vi "Move to Named Position (Sub VI).vi"(10 "named_position":T1, 11 "_num_axes":i32) -> (0 "error out":errorcluster)   [LabVIEW 2020, in "Manipulator.lvlib"]
uses:
  Manipulator.lvlib
  Settings/Named Position.ctl
  Manipulator-CLIDriver/Manipulator CLI Driver.lvlib
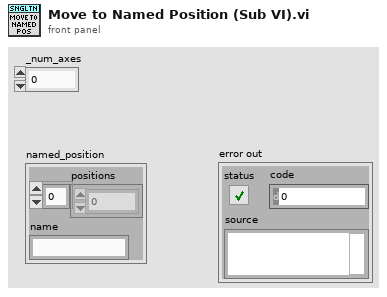
[diagram p1: front panel]
types:
  T1 = typedef "Manipulator.lvlib/Named Position.ctl" = cluster{"positions":dbl[], "name":string}
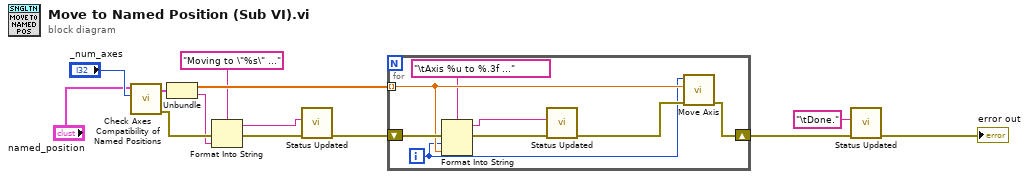
[diagram p0: block diagram]
diagram:
  n1 = call "Check Axes Compatibility of Named Positions.vi"("Num Axes"="_num_axes", "named_position"="named_position") -> ("error out"=w12:errorcluster, "named_position"=w11:T1)  [unwired: 8 in]
  n2 = Unbundle(w11) -> ("positions"=w8:dbl[], "name"=w4:string)
  n3 = Format Into String(format string="Moving to \"%s\" ...", error in=w12, w4) -> (resulting string=w5:string, error out=w7:errorcluster)  [unwired: 1 in]
  n4 = call "Status Updated.vi"("error in (no error)"=w7, "Status"=w5) -> ("error out"=w6:errorcluster)  [unwired: 9 in]
  n5 = for {
    tunnel: w8 -> [w16] mode=indexing
    shift-right: [w21] -> w9
    shift-left: w6 -> [w20]
    i -> [w15]
    n6 = Format Into String(format string="\tAxis %u to %.3f ...", error in=w20, w15, w16) -> (resulting string=w17:string, error out=w19:errorcluster)  [unwired: 1 in]
    n7 = call "Status Updated.vi"("error in (no error)"=w19, "Status"=w17) -> ("error out"=w18:errorcluster)  [unwired: 9 in]
    n8 = call "Move Axis.vi"("error in (no error)"=w18, "Position"=w16, "Axis"=w15) -> ("error out"=w21:errorcluster)  [unwired: 8 in]
  }
  n9 = call "Status Updated.vi"("error in (no error)"=w9, "Status"="\tDone.") -> ("error out"=→"error out":errorcluster)  [unwired: 9 in]
